vi "Entry.vi"(8 "error in (no error)":errorcluster, 11 "New State":refnum<class "Announcing.lvclass">) -> (0 "error out":errorcluster, 3 "State out":refnum<class "Announcing.lvclass">)   [LabVIEW 2013, in "Receiver.lvlib" / "Receiver Commands Using Processor.lvlib" / "Connect Command.lvlib" / "Announcing.lvclass"]
doc: "This is an abstract method. Override this method to define the behavior when you enter the state."
uses:
  Announcing.lvclass
  Receiver Messages/Annouce Msg/Annouce Msg.lvclass
  <vilib>/ActorFramework/Actor/Actor.lvclass/Actor.ctl
  <vilib>/ActorFramework/Message Enqueuer/Message Enqueuer.lvclass/Message Enqueuer.ctl
  Receiver Messages/Annouce Msg/Annouce Msg.lvclass/Annouce Msg.ctl
  Announcing.lvclass/Announcing.ctl
  Connect Command.lvclass
  <vilib>/ActorFramework/Message Enqueuer/Init from Existing Queue.vi
  <vilib>/ActorFramework/Message Enqueuer/Enqueue.vi
  <vilib>/ActorFramework/Message Priority Queue/Priority Enqueue.vi
  <vilib>/ActorFramework/Message Enqueuer/Message Enqueuer.lvclass
  <vilib>/ActorFramework/Actor/Actor.lvclass
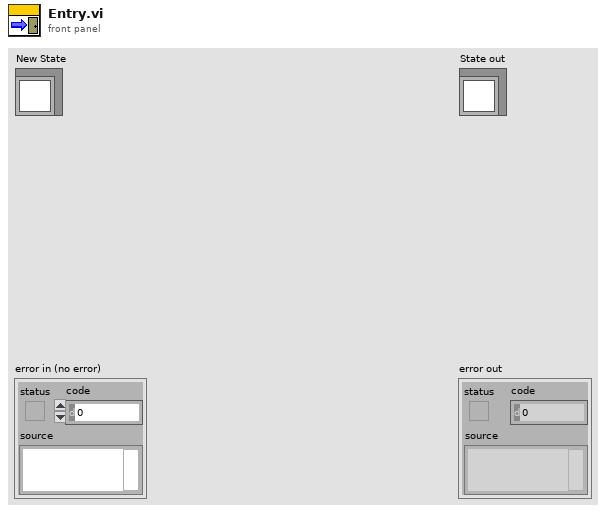
[diagram p1: front panel]
types:
  T1 = typedef "Command Processor.lvlib/Command.lvlib/Command.lvclass/Command Status.ctl" = cluster{"Command Name":string, "Current State Status":T2, "Command Start Time":timestamp, "Command End Time":timestamp, "Previous State Status":T2}
  T2 = typedef "Command Processor.lvlib/Command.lvlib/Command.lvclass/State Status.ctl" = cluster{"State Name":string, "State Entry Time":timestamp, "State Exit Time":timestamp}
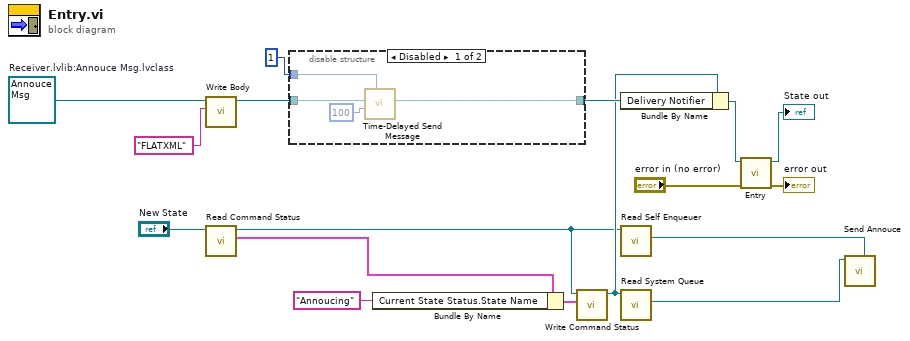
[diagram p0: block diagram]
diagram:
  w7 = refnum<class "Annouce Msg.lvclass"> refnum  # Receiver.lvlib:Annouce Msg.lvclass
  n1 = call-dynamic "Write Body.vi"("Body"="FLATXML", "Annouce Msg in"=w7) -> ("Annouce Msg out"=w6:refnum<class "Annouce Msg.lvclass">)  [unwired: 8 in, 1 out]
  n2 = call-dynamic "Read Command Status.vi"("Command in"="New State") -> ("Command Status"=w11:T1, "Command out"=w2:refnum<class "Announcing.lvclass">)  [unwired: 8 in, 1 out]
  n3 = disable-structure shown="Disabled" {
    disable-tunnel: [w21 _] -> w13
    disable-tunnel: w6 -> [w19 _]
    disable-tunnel: u32 1 ("# Copies (0 = infinite repeat)") -> [w18 _]
    frame Disabled {
      n4 = call <vilib>:"Time-Delayed Send Message.vi"("# Copies (0 = infinite repeat)"=w18, "Milliseconds To Wait"=100, "Message"=w19) -> ("Delivery Notifier"=w21:refnum<notifier>)  [unwired: 7 in, 1 out]
    }
    frame Enabled {
    }
  }
  n5 = Bundle By Name(cluster=w11, "Current State Status.State Name"="Annoucing") -> (w10:T1)
  n6 = call-dynamic "Write Command Status.vi"("Command Status"=w10, "Command in"=w2) -> ("Command out"=w8:refnum<class "Announcing.lvclass">)  [unwired: 8 in, 1 out]
  n7 = Bundle By Name(cluster=w8, "Delivery Notifier"=w13) -> (w14:refnum<class "Announcing.lvclass">)
  n8 = call <vilib>:"Read Self Enqueuer.vi"("Actor"=w2) -> ("Self Enqueuer"=w1:refnum<class "Message Enqueuer.lvclass">)  [unwired: 10 in]
  n9 = call-dynamic "Read System Queue.vi"("Command in"=w8) -> ("Actor Framework:Message Enqueuer"=w3:refnum<class "Message Enqueuer.lvclass">)  [unwired: 8 in, 2 out]
  n10 = call-parent "Entry.vi"("error in (no error)"="error in (no error)", "New State"=w14) -> ("error out"=→"error out":errorcluster, "State out"=→"State out":refnum<class "Announcing.lvclass">)  [unwired: 8 in]
  n11 = call "Send Annouce.vi"("Command Queue"=w1, "Message Enqueuer"=w3) -> ()  [unwired: 8 in, 2 out]
